vi "START5Fancy.vi"() -> ()   [LabVIEW 2024]
uses:
  <vilib>/Utility/file.llb/Read Delimited Spreadsheet (DBL).vi
panel:
  in  "stop":bool
  in  "Numeric 2":dbl
  in  "Numeric":dbl
  out "Waveform Chart 3":dbl[](graph)
  out "Waveform Chart 2":dbl[](graph)
  out "Flow Rate":dbl[](graph)
  in  "Color Box":u32(colorbox)
  # "Flow Rate of"
  # "Flow Rate of"
  # "Flow Rate of"
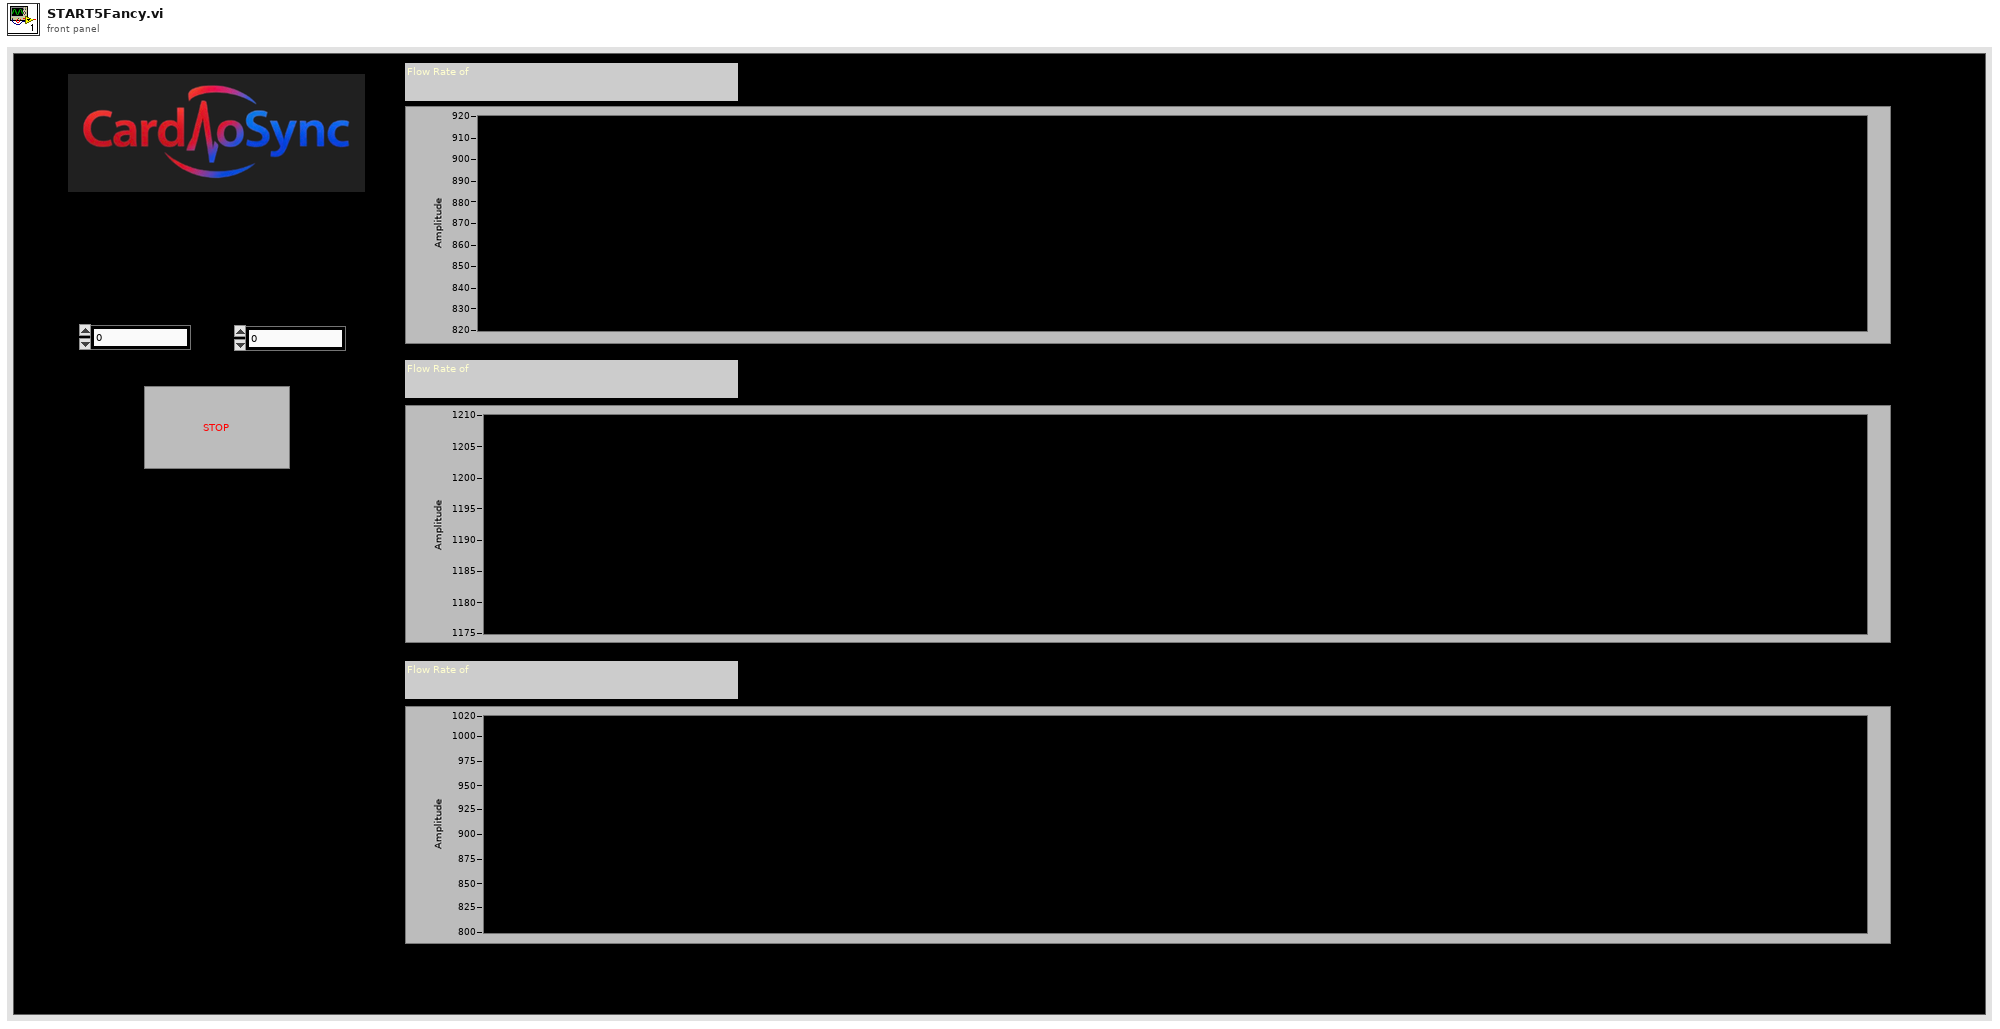
[diagram p1: front panel]
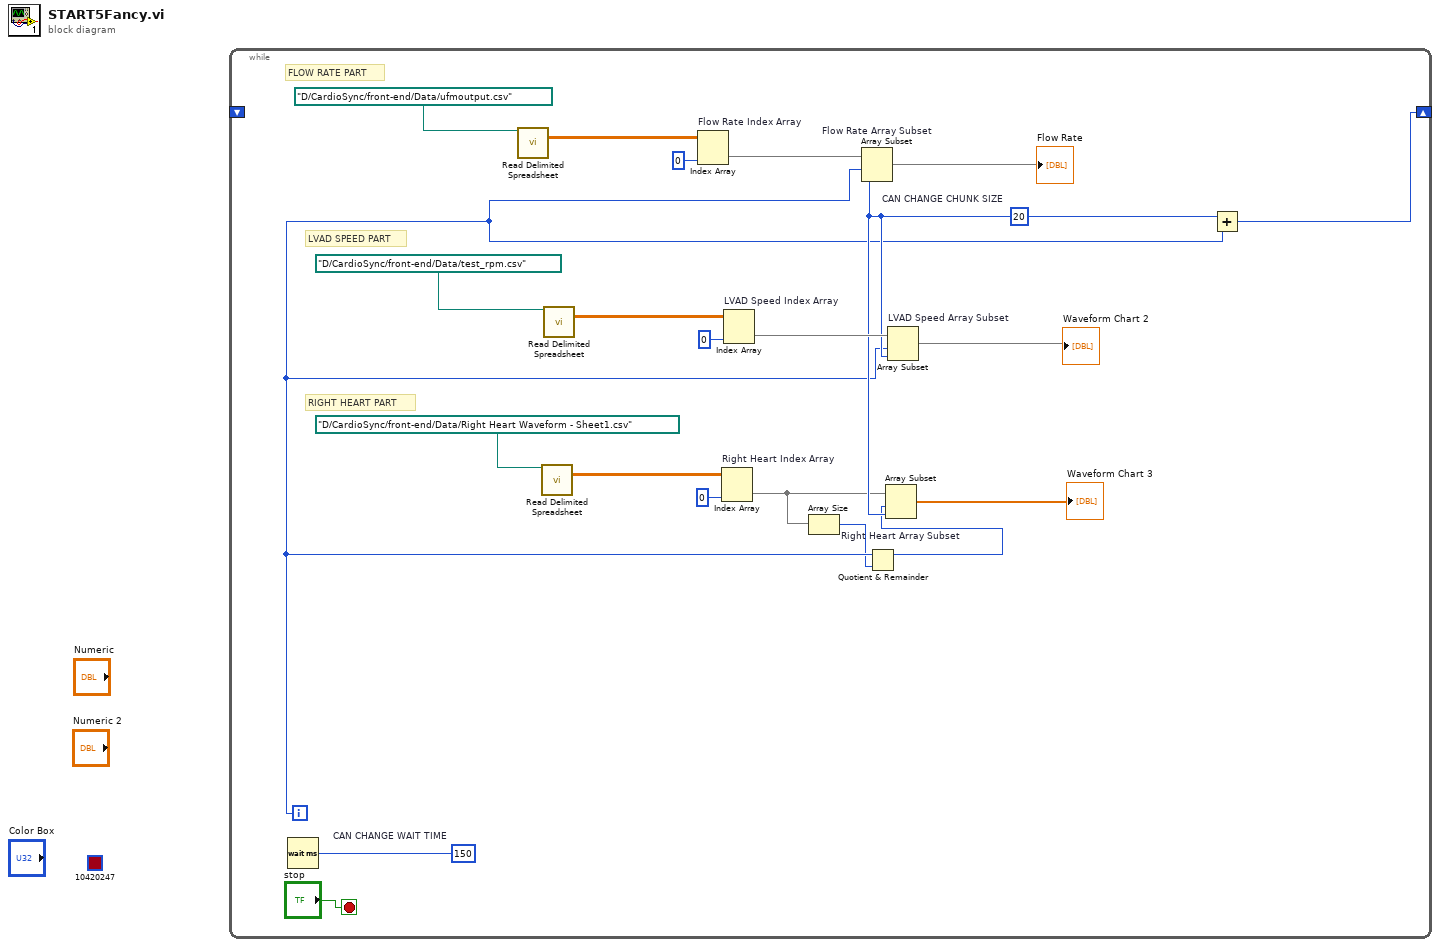
[diagram p0: block diagram]
diagram:
  (unwired) u32 10420247 ("Color Box 2")
  n1 = while {
    shift-right: [w17] -> _
    shift-left: _ -> [_]
    i -> [w3]
    stop <- "stop" stop-if-true
    w18 = u32 150  # CAN CHANGE WAIT TIME
    w10 = 20  # CAN CHANGE CHUNK SIZE
    # "RIGHT HEART PART"
    # "LVAD SPEED PART"
    # "FLOW RATE PART"
    n2 = Wait (ms)(milliseconds to wait=w18) -> ()  [unwired: 1 out]
    n3 = call-poly <vilib>:"Read Delimited Spreadsheet.vi"("file path (dialog if empty)"=path "D:/CardioSync/front-end/Data/ufmoutput.csv") -> ("all rows"=w20:dbl[][])  [unwired: 9 in, 5 out]
    n4 = call-poly <vilib>:"Read Delimited Spreadsheet.vi"("file path (dialog if empty)"=path "D:/CardioSync/front-end/Data/Right Heart Waveform - Sheet1.csv") -> ("all rows"=w11:dbl[][])  [unwired: 9 in, 5 out]
    n5 = call-poly <vilib>:"Read Delimited Spreadsheet.vi"("file path (dialog if empty)"=path "D:/CardioSync/front-end/Data/test_rpm.csv") -> ("all rows"=w14:dbl[][])  [unwired: 9 in, 5 out]
    n6 = Index Array "Flow Rate Index Array"(array=w20, index (col)=0 ("disabled index (col)")) -> (element=w19:dbl[])  [unwired: 1 in]
    n7 = Index Array "Right Heart Index Array"(array=w11, index (col)=0 ("disabled index (col)")) -> (element=w4:dbl[])  [unwired: 1 in]
    n8 = Index Array "LVAD Speed Index Array"(array=w14, index (col)=0 ("disabled index (col)")) -> (element=w13:dbl[])  [unwired: 1 in]
    n9 = Array Size(array=w4) -> (size(s)=w2:i32)
    n10 = Array Subset "Flow Rate Array Subset"(array=w19, index=w3, length=w10) -> (→"Flow Rate":dbl[])
    n11 = Quotient & Remainder(x=w3, y=w2) -> (x-y*floor(x/y)=w1:i32)  [unwired: 1 out]
    n12 = Array Subset "Right Heart Array Subset"(array=w4, index=w1, length=w10) -> (→"Waveform Chart 3":dbl[])
    n13 = Array Subset "LVAD Speed Array Subset"(array=w13, index=w3, length=w10) -> (→"Waveform Chart 2":dbl[])
    n14 = Add(x=w10, y=w3) -> (x+y=w17:i32)
  }
